vi "Lab6.vi"() -> ()   [LabVIEW 2021]
panel:
  out "RecvValue8":dbl
  out "RecvValue7":dbl
  out "RecvValue6":dbl
  out "RecvValue5":dbl
  out "RecvValue4":dbl
  out "RecvValue3":dbl
  out "Y":dbl
  out "X":dbl
  in  "SendValue8":dbl
  in  "SendValue7":dbl
  in  "SendValue6":dbl
  in  "SendValue5":dbl
  in  "SendValue4":dbl
  in  "SendValue3":dbl
  in  "SendValue2":dbl
  in  "SendValue1":dbl
  in  "Send Button":bool
  in  "stop":bool
  in  "Size of Rectangle":i16
  in  "Display History":bool
  out "2D Picture":picture
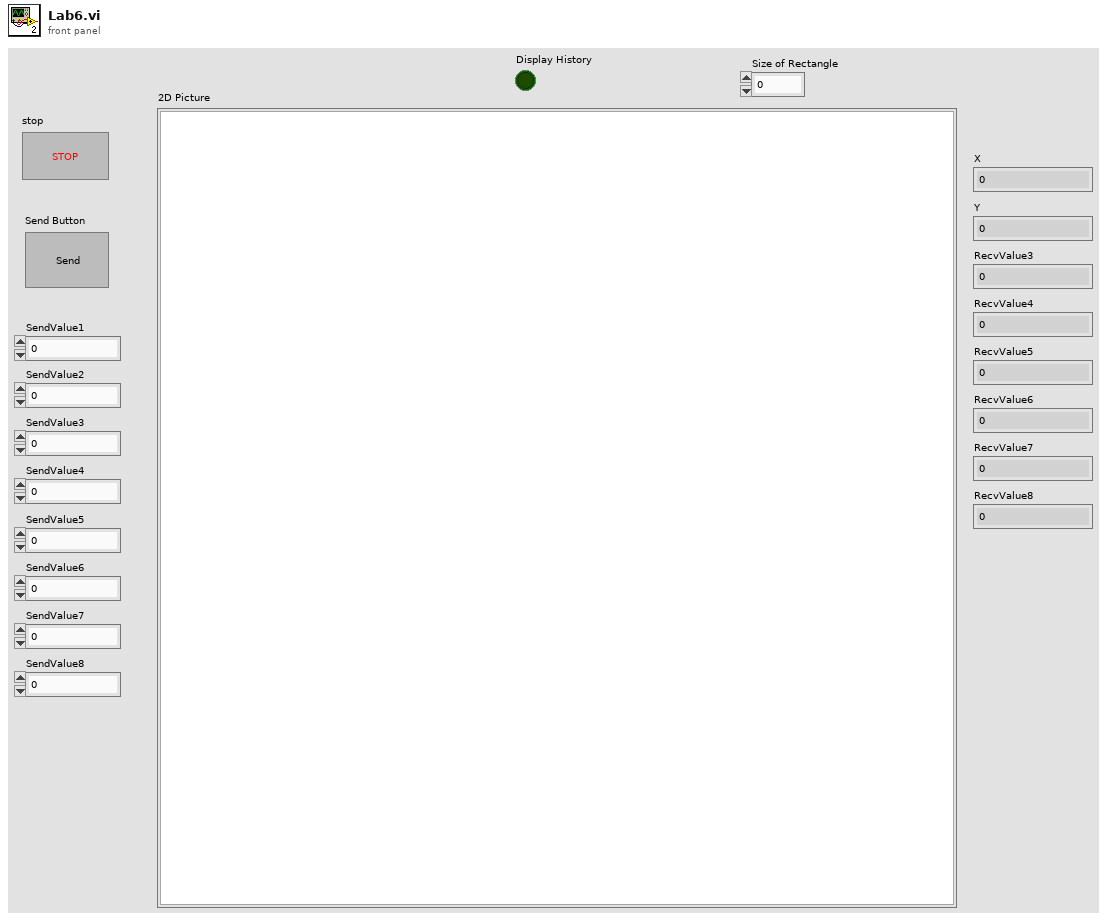
[diagram p1: front panel]
types:
  T1 = enum16{"Standard", "Buffered", "CRLF", "Immediate"}
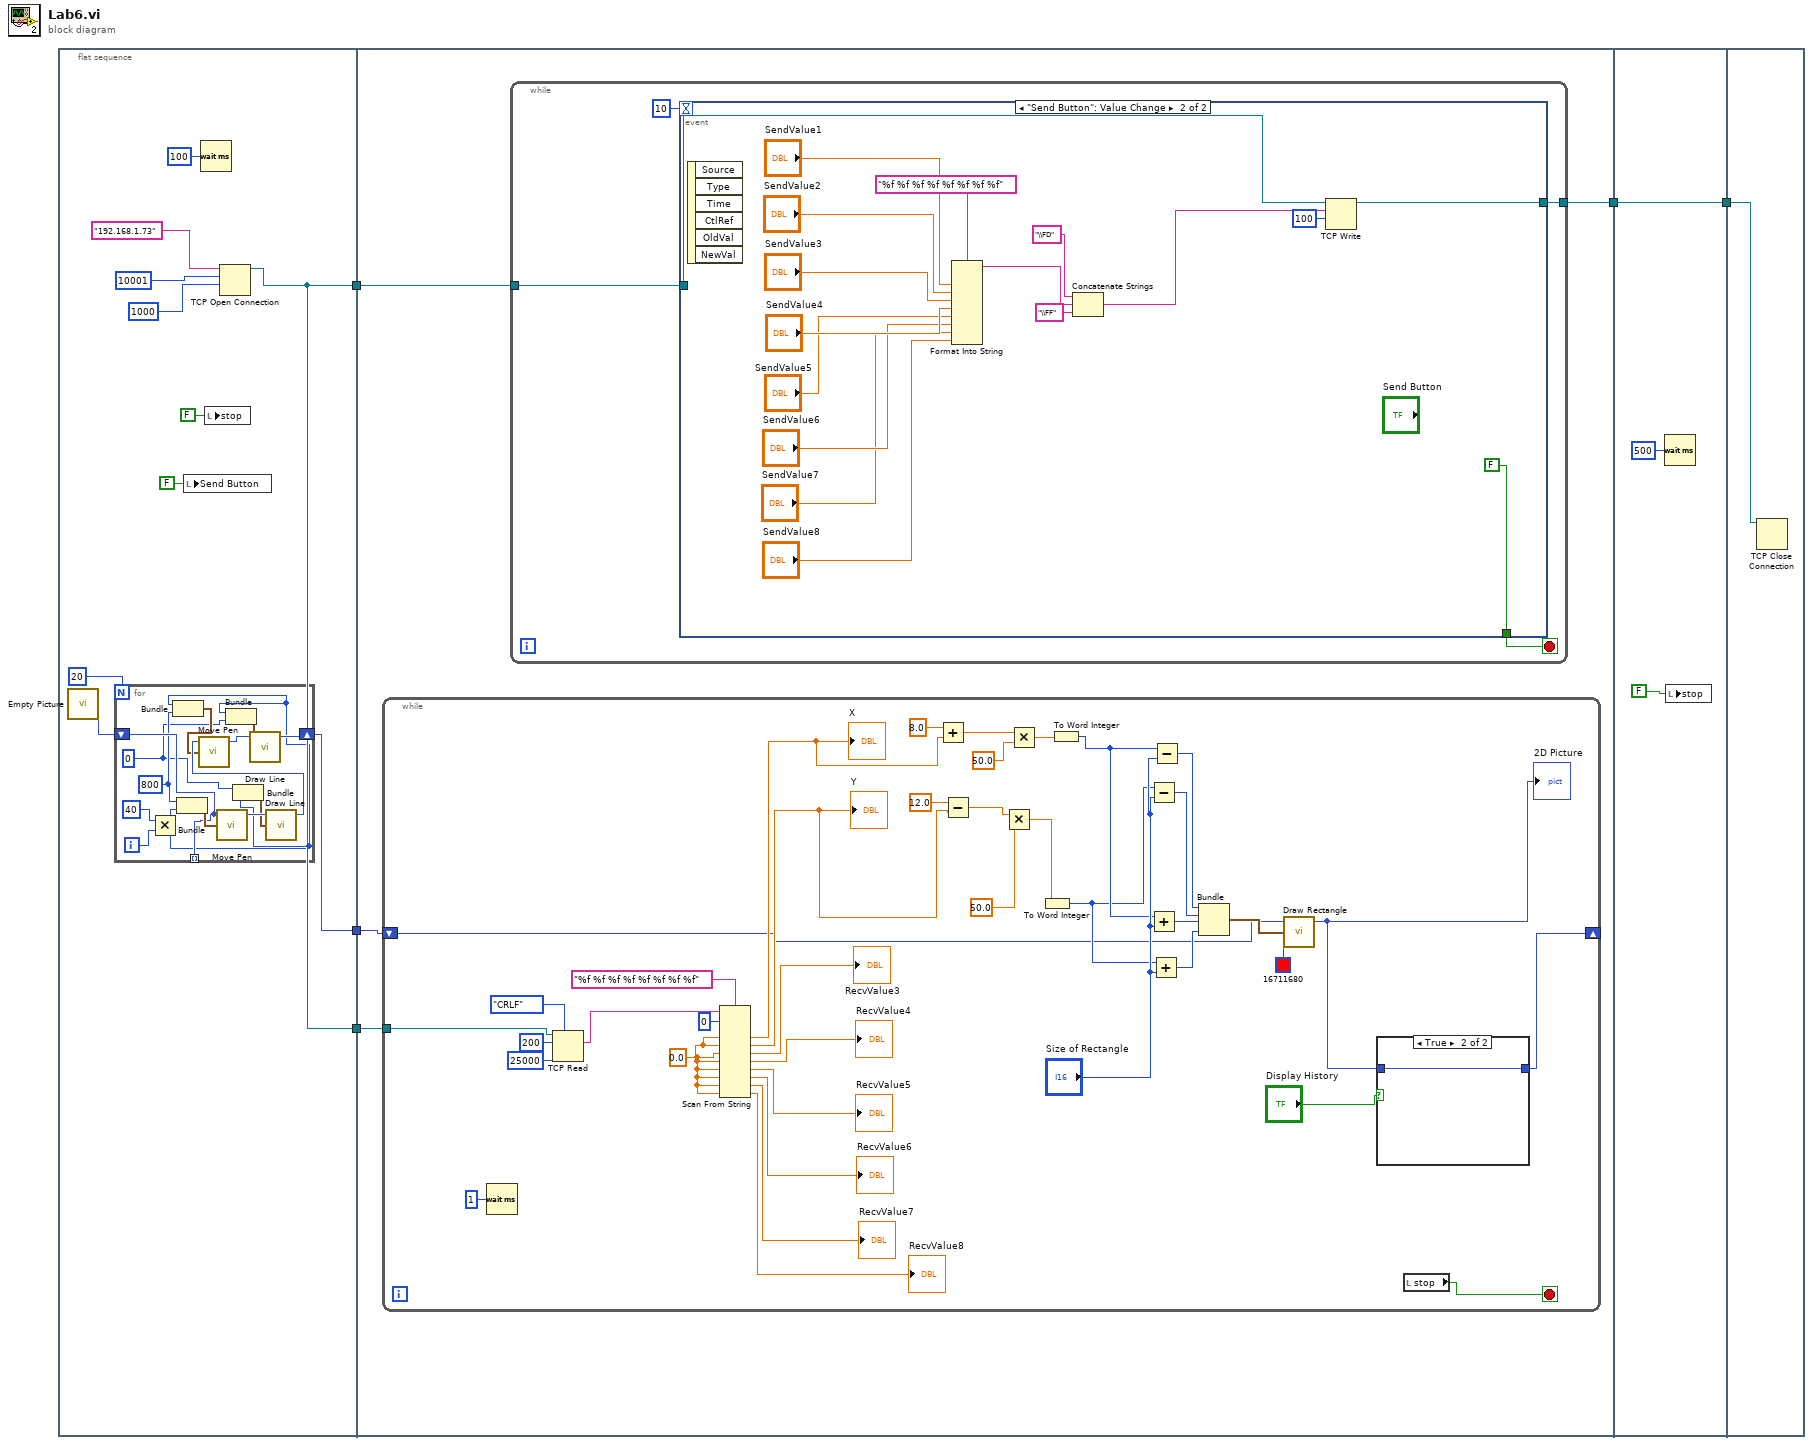
[diagram p0: block diagram]
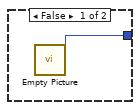
[diagram p2: hidden frame]
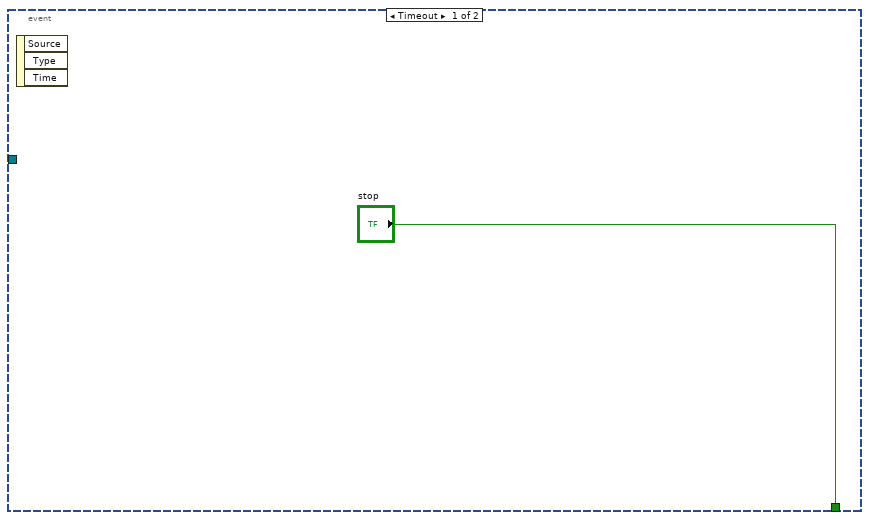
[diagram p3: hidden frame]
diagram:
  n1 = flat-sequence {
    tunnel: [w6] -> w5
    tunnel: [w9] -> w4
    tunnel: [w9] -> w1
    tunnel: w5 -> [w33]
    tunnel: w4 -> [w32]
    tunnel: [w31] -> w2
    tunnel: w1 -> [w30]
    tunnel: [w99] -> w3
    tunnel: w2 -> [w99]
    tunnel: w3 -> [w100]
    frame #0 {
      n2 = call "Empty Picture"() -> ("empty picture"=w7:picture)
      n3 = for {
        N: 20 -> [_]
        tunnel: [w22] -> _ mode=indexing
        shift-right: [w23] -> w6
        shift-left: w7 -> [w22]
        i -> [w27]
        w20 = 800
        w18 = 0
        n4 = Multiply(x=40, y=w27) -> (x*y=w17:i32)
        n5 = Bundle(w17, w20) -> (w19:cluster{i32, i32})  [unwired: 1 in]
        n6 = Bundle(w20, w17) -> (w25:cluster{i32, i32})  [unwired: 1 in]
        n7 = call <vilib>:"Move Pen.vi"("new position"=w25, "picture"=w22) -> ("new picture"=w29:picture)  [unwired: 3 in]
        n8 = Bundle(w17, w18) -> (w16:cluster{i32, i32})  [unwired: 1 in]
        n9 = Bundle(w18, w17) -> (w21:cluster{i32, i32})  [unwired: 1 in]
        n10 = call <vilib>:"Draw Line.vi"("picture"=w29, "end point"=w21) -> ("new picture"=w26:picture)  [unwired: 7 in]
        n11 = call <vilib>:"Move Pen.vi"("new position"=w19, "picture"=w26) -> ("new picture"=w24:picture)  [unwired: 3 in]
        n12 = call <vilib>:"Draw Line.vi"("picture"=w24, "end point"=w16) -> ("new picture"=w23:picture)  [unwired: 7 in]
      }
      n13 = local write "Send Button"(FALSE ("Send Button")) -> ()
      n14 = Wait (ms)(milliseconds to wait=u32 100) -> ()  [unwired: 1 out]
      n15 = local write "stop"(FALSE ("stop")) -> ()
      n16 = TCP Open Connection(address="192.168.1.73", remote port or service name=u16 10001, timeout ms (60000)=1000) -> (connection ID=w9:refnum<k5>)  [unwired: 2 in, 1 out]
    }
    frame #1 {
      n17 = while {
        shift-right: [w71] -> _
        shift-left: w33 -> [w35]
        tunnel: w30 -> [w65]
        stop <- w70 stop-if-true
        w61 = 0.0 ("default value 1")
        n18 = Wait (ms)(milliseconds to wait=u32 1) -> ()  [unwired: 1 out]
        n19 = TCP Read(connection ID=w65, bytes to read=200, 7:T1."CRLF" ("mode (standard)"), 9:25000 ("timeout ms (25000)")) -> (data out=w64:string)  [unwired: 1 in, 2 out]
        n20 = Scan From String(format string="%f %f %f %f %f %f %f %f", input string=w64, initial scan location=u32 0, default 1=w61, default 2=w61, default 3=w61, default 4=w61, default 5=w61, default 6=w61, default 7=w61, default 8=w61) -> (output 1=w51:dbl, output 2=w52:dbl, output 3=→"RecvValue3":dbl, output 4=→"RecvValue4":dbl, output 5=→"RecvValue5":dbl, output 6=→"RecvValue6":dbl, output 7=→"RecvValue7":dbl, output 8=→"RecvValue8":dbl)  [unwired: 1 in, 3 out]
        "X" <- w51
        "Y" <- w52
        n21 = Add(x=8.0, y=w51) -> (x+y=w49:dbl)
        n22 = Subtract(x=12.0, y=w52) -> (x-y=w47:dbl)
        n23 = Multiply(x=w47, y=50.0) -> (x*y=w45:dbl)
        n24 = Multiply(x=w49, y=50.0) -> (x*y=w46:dbl)
        n25 = To Word Integer(number=w45) -> (16bit integer=w42:i16)
        n26 = To Word Integer(number=w46) -> (16bit integer=w43:i16)
        n27 = Subtract(x=w42, y="Size of Rectangle") -> (x-y=w39:i16)
        n28 = Add(x=w43, y="Size of Rectangle") -> (x+y=w41:i16)
        n29 = Add(x=w42, y="Size of Rectangle") -> (x+y=w40:i16)
        n30 = Subtract(x=w43, y="Size of Rectangle") -> (x-y=w38:i16)
        n31 = Bundle(w38, w39, w41, w40) -> (w37:cluster{i16, i16, i16, i16})  [unwired: 1 in]
        n32 = call <vilib>:"Draw Rectangle.vi"("picture"=w35, "rect"=w37, "color(black)"=u32 16711680) -> ("new picture"=w34:picture)  [unwired: 6 in]
        "2D Picture" <- w34
        n33 = case shown="True" "Display History" {
          tunnel: w34 -> [_ w74]
          tunnel: [w73 w74] -> w71
          frame False {
            n34 = call "Empty Picture"() -> ("empty picture"=w73:picture)
          }
          frame True {
          }
        }
        n35 = local read "stop"() -> (w70:bool)
      }
      n36 = while {
        tunnel: w32 -> [w76]
        tunnel: [w75] -> w31
        stop <- w77 stop-if-true
        n37 = event shown="[1] \"Send Button\": Value Change" {
          selector: _ -> [_ _]
          dyn-events: _ -> [_ _]
          timeout: 10 -> [_ _]
          tunnel: ["stop" FALSE] -> w77
          tunnel: w76 -> [_ w95]
          tunnel: [_ w80] -> w75
          event Timeout {
            n38 = event-data() -> ()  [unwired: 1 in, 3 out]
          }
          event "Send Button": Value Change {
            n39 = event-data() -> ()  [unwired: 1 in, 6 out]
            n40 = Format Into String(format string="%f %f %f %f %f %f %f %f", "SendValue1", "SendValue2", "SendValue3", "SendValue4", "SendValue5", "SendValue6", "SendValue7", "SendValue8") -> (resulting string=w85:string)  [unwired: 2 in, 1 out]
            n41 = Concatenate Strings("\\FD" ("string"), w85, "\\FF" ("string")) -> (w82:string)
            n42 = TCP Write(connection ID=w95, data in=w82, 9:100 ("timeout ms (25000)")) -> (connection ID out=w80:refnum<k5>)  [unwired: 1 in, 2 out]
          }
        }
      }
    }
    frame #2 {
      n43 = Wait (ms)(milliseconds to wait=u32 500) -> ()  [unwired: 1 out]
      n44 = local write "stop"(FALSE ("stop")) -> ()
    }
    frame #3 {
      n45 = TCP Close Connection(connection ID=w100) -> ()  [unwired: 2 in, 2 out]
    }
  }
